vi "Connect.vi"(8 "error in":errorcluster, 11 "2936r in":refnum<class "2936r.lvclass">) -> (0 "error out":errorcluster, 3 "2936r out":refnum<class "2936r.lvclass">)   [LabVIEW 2018, in "2936r.lvlib" / "2936r.lvclass"]
uses:
  2936r.lvclass
  2936r.lvclass/2936r.ctl
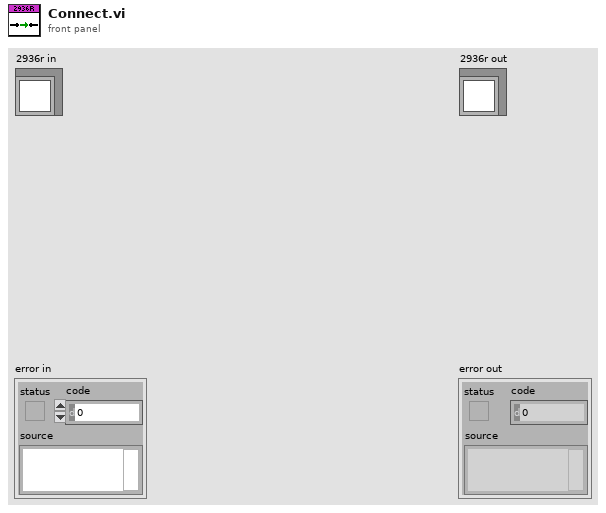
[diagram p1: front panel]
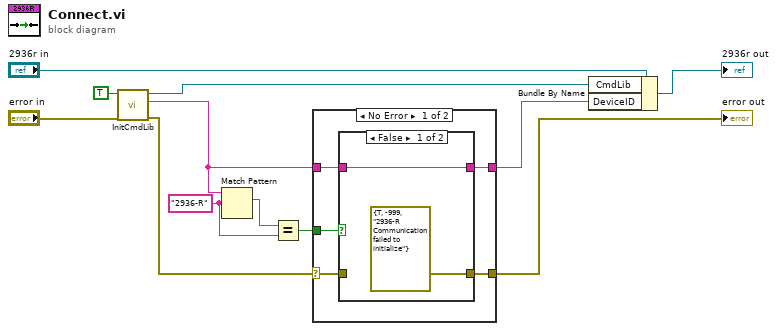
[diagram p0: block diagram]
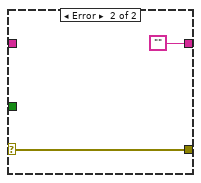
[diagram p3: hidden frame]
diagram:
  w7 = "2936-R" ("regular expression")
  n1 = call <instrlib>:"InitCmdLib.vi"("error in (no error)"="error in", "logging"=TRUE) -> ("error out"=w1:errorcluster, "Device Key"=w5:string, "CmdLib"=w2:refnum<k24>)  [unwired: 7 in]
  n2 = Match Pattern(string=w5, regular expression=w7) -> (match substring=w8:string)  [unwired: 1 in, 3 out]
  n3 = Equal?(x=w8, y=w7) -> (x = y?=w6:bool)
  n4 = case shown="No Error" w1 {
    selector: w1 -> [w13 w23]
    tunnel: w6 -> [w17 _]
    tunnel: w5 -> [w16 _]
    tunnel: [w15 ""] -> w4
    tunnel: [w14 w23] -> w3
    frame No Error {
      n5 = case shown="False" w17 {
        tunnel: w16 -> [w19 w21]
        tunnel: [w19 w21] -> w15
        tunnel: w13 -> [_ w20]
        tunnel: [errorcluster {"status"=TRUE, "code"=-999, "source"="2936-R Communication failed to initialize"} ("error out") w20] -> w14
        frame False {
        }
        frame True {
        }
      }
    }
    frame Error {
    }
  }
  "error out" <- w3
  n6 = Bundle By Name(cluster="2936r in", "CmdLib"=w2, "DeviceID"=w4) -> (→"2936r out":refnum<class "2936r.lvclass">)
